vi "Query Output State.vi"(8 "error in (no error)":errorcluster {"code" format="%.0x"}, 9 "Output State (0: Constant Voltage)":i32(ring) items=["Constant Voltage"=0, "Constant Current"=1, "Unregulated"=4, "Over Voltage"=2, "Over Current"=3], 10 "Channel Name (1)":string="1", 11 "VISA resource name":refnum<visa-resource-name>) -> (0 "error out":errorcluster {"code" format="%.0x"}, 2 "In State":bool, 3 "VISA resource name out":refnum<visa-resource-name>)   [LabVIEW 2014, in "Agilent N6700 Series.lvlib"]
doc: "Returns whether the power supply is in a particular output state.\n\nA constant voltage condition occurs when the output voltage is equal to the value of Level in <B>Configure Voltage Level.vi</B> and the current is less than or equal to the value of Limit in <B>Configure Current Limit.vi</B>.\n\nA constant current condition occurs when the output current is equal to the value of Limit in <B>Configure Current Limit.vi</B> and Behavior in <B>Configure Current Limit.vi</B> is set to Regulatory Limit.\n\nAn unregulated condition occurs when the output voltage is less than the value of Level in <B>Configure Voltage Level.vi</B> and the current is less than the value of Limit in <B>Configure Current Limit.vi</B>.\n\nAn over-voltage condition occurs when the output voltage is equal to or greater than the value of Limit in <B>Configure Over Voltage Protection.vi</B>.\n\nAn over-current condition occurs when the output current is equal to or greater than the value of Limit in <B>Configure Current Limit.vi</B> and Behavior in <B>Configure Current Limit.vi</B> is set to Trip Limit.\n\nWhen either an over-voltage condition or an over-current condition occurs, the power supply's output protection disables the output. If the power supply is in an over-voltage or over-current state, it does not produce power until the output protection is reset. The <B>Reset Output Protection.vi</B> resets the output protection. Once the output protection is reset, the power supply resumes generating a power signal."
uses:
  Agilent N6700 Series.lvlib
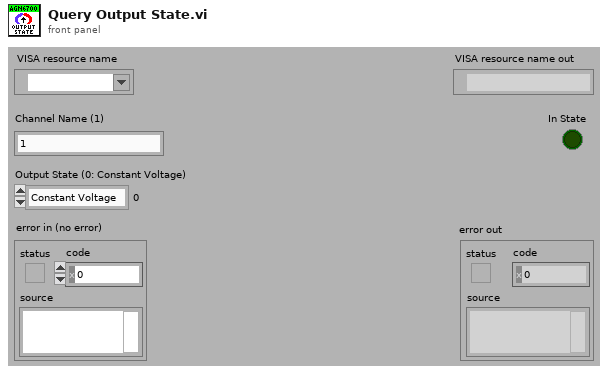
[diagram p1: front panel]
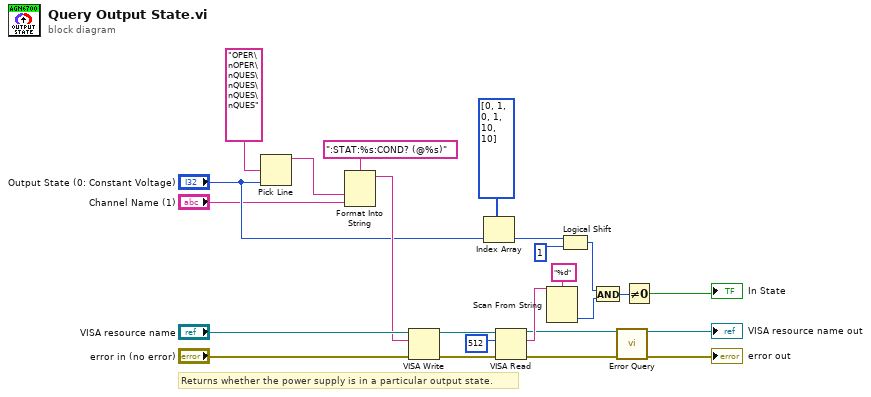
[diagram p0: block diagram]
diagram:
  # "Returns whether the power supply is in a particular output state."
  n1 = Pick Line(multi-line string="OPER\nOPER\nQUES\nQUES\nQUES\nQUES", line index="Output State (0: Constant Voltage)") -> (output string=w17:string)  [unwired: 1 in]
  n2 = Format Into String(format string=":STAT:%s:COND? (@%s)", w17, "Channel Name (1)") -> (resulting string=w14:string)  [unwired: 2 in, 1 out]
  n3 = VISA Write(VISA resource name="VISA resource name", write buffer=w14, error in (no error)="error in (no error)") -> (VISA resource name out=w23:refnum<visa-resource-name>, error out=w22:errorcluster)  [unwired: 1 out]
  n4 = Index Array(array=i32[] [0, 1, 0, 1, 10, 10], index="Output State (0: Constant Voltage)") -> (element=w3:i32)
  n5 = VISA Read(VISA resource name=w23, byte count=u32 512, error in (no error)=w22) -> (VISA resource name out=w5:refnum<visa-resource-name>, read buffer=w21:string, error out=w4:errorcluster)  [unwired: 1 out]
  n6 = Scan From String(format string="%d", input string=w21) -> (output 1=w11:i32)  [unwired: 3 in, 3 out]
  n7 = Logical Shift(y=w3, x=1) -> (x << y=w1:i32)
  n8 = And(x=w1, y=w11) -> (x .and. y?=w9:i32)
  n9 = call "Error Query.vi"("VISA resource name"=w5, "error in (no error)"=w4) -> ("VISA resource name out"=→"VISA resource name out":refnum<visa-resource-name>, "error out"=→"error out":errorcluster)  [unwired: 10 in, 2 out]
  n10 = Not Equal To 0?(x=w9) -> (x != 0?=→"In State":bool)
